vi "Init Message Transport Queue.vi"(6 "Max Queue Size":i32=-1, 8 "error in (no error)":errorcluster, 11 "Message":refnum<class "Message Interface.lvclass">) -> (0 "error out":errorcluster, 3 "Message Transport Queue out":refnum<class "Message Transport Queue.lvclass">)   [LabVIEW 2016, in "Stream Mediator.lvlib" / "Message Transport Queue.lvclass"]
doc: "--\nCopyright © 2017 Composed SystemsI All rights reserved.\n\nAuthor: Jon McBee <jon.mcbee@composed.io>\n\nThis library is provided \"AS IS\" ,WITHOUT WARRANTIES OR\nCONDITIONS OF ANY KIND, either express or implied.\n\nComposed Systems -- composed.io\n\nStream 0.0.1.1\nJon McBee - Composed Systems\nCopyright (c) 2017, Composed Systems"
uses:
  <userlib>/Composed Systems/Stream/Mediator/Classes/Message Transport Queue/Message Transport Queue.lvclass
  <userlib>/Composed Systems/Stream/Mediator/Classes/Message Interface/Message Interface.lvclass
  <userlib>/Composed Systems/Stream/Mediator/Classes/Message Transport Queue/Message Transport Queue.lvclass/Message Transport Queue.ctl
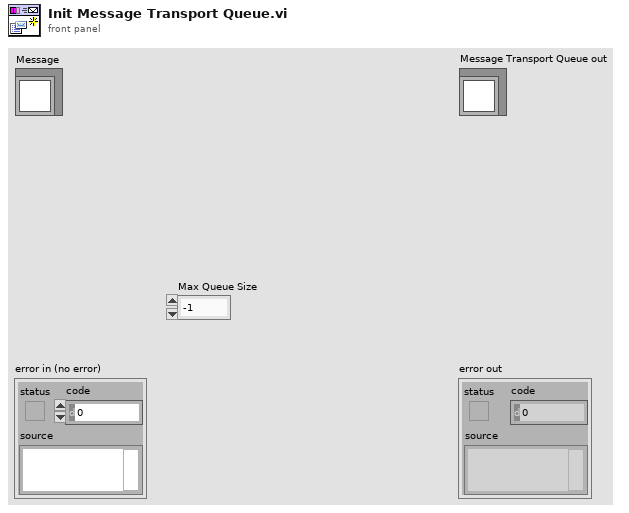
[diagram p1: front panel]
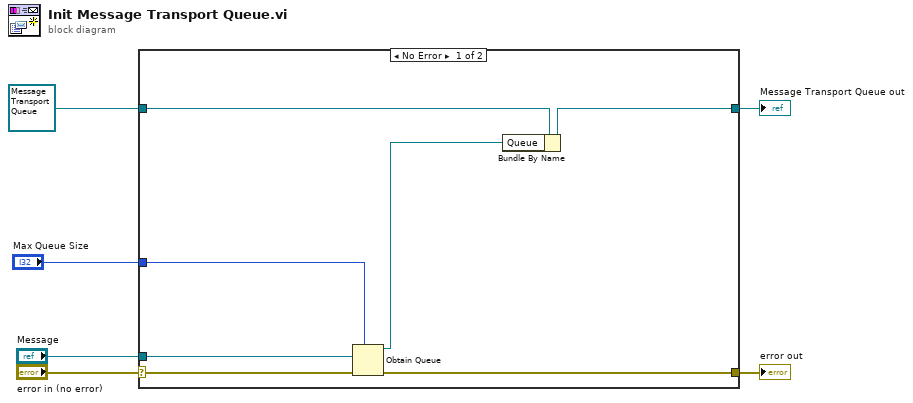
[diagram p0: block diagram]
diagram:
  n1 = case shown="No Error" "error in (no error)" {
    selector: "error in (no error)" -> [w13 w15]
    tunnel: [w12 w15] -> w5
    tunnel: [w10 w14] -> w3
    tunnel: refnum<class "Message Transport Queue.lvclass"> refnum ("Message Transport Queue in") -> [w11 w14]
    tunnel: "Max Queue Size" -> [w8 _]
    tunnel: "Message" -> [w7 _]
    frame No Error {
      n2 = Obtain Queue(max queue size (-1, unlimited)=w8, element data type=w7, error in (no error)=w13) -> (queue out=w9:refnum<queue>, error out=w12:errorcluster)  [unwired: 2 in, 1 out]
      n3 = Bundle By Name(cluster=w11, "Queue"=w9) -> (w10:refnum<class "Message Transport Queue.lvclass">)
    }
    frame Error {
    }
  }
  "error out" <- w5
  "Message Transport Queue out" <- w3
